vi "test_TCP_2_ Host.vi"() -> ()   [LabVIEW 2014]
panel:
  out "output array":string[](array[string])
  out "output_strCmd":string
  out "output_strAccum":string
  out "error out":errorcluster
  in  "stop":bool
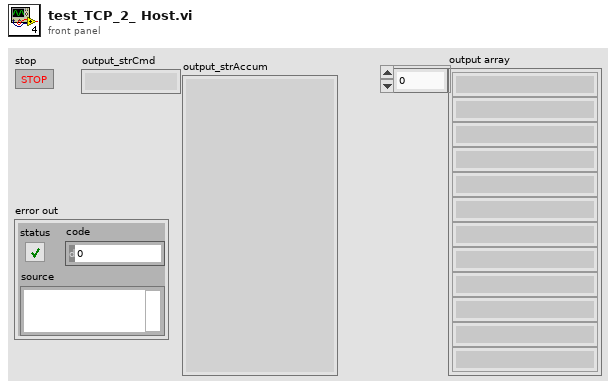
[diagram p1: front panel]
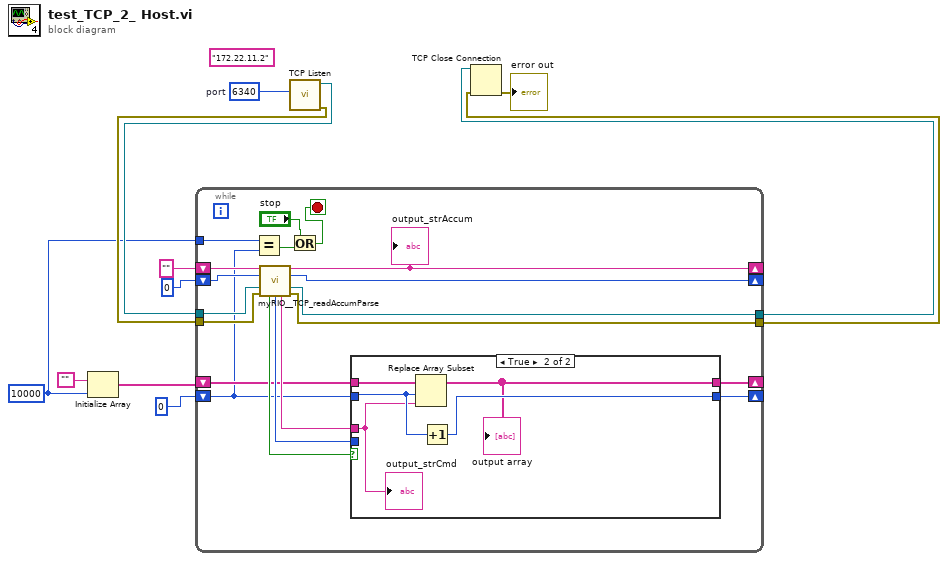
[diagram p0: block diagram]
diagram:
  w1 = 10000 ("dimension size")
  (unwired) "172.22.11.2" ("address")
  w8 = u16 6340  # port
  n1 = Initialize Array("", w1) -> (w2:string[])
  n2 = call <vilib>:"TCP Listen.vi"("port"=w8) -> ("error out"=w6:errorcluster, "connection ID"=w7:refnum<k5>)  [unwired: 6 in, 3 out]
  n3 = while {
    tunnel: w7 -> [w31]
    tunnel: [w28] -> w10
    shift-right: [w26] -> _
    shift-left: "" -> [w29]
    tunnel: w6 -> [w30]
    tunnel: [w27] -> w11
    shift-right: [w24] -> _
    shift-left: 0 -> [w25]
    shift-right: [w19] -> _
    shift-left: w2 -> [w20]
    shift-right: [w18] -> _
    shift-left: 0 -> [w13]
    tunnel: w1 -> [w14]
    stop <- w15 stop-if-true
    n4 = Equal?(x=w14, y=w13) -> (x = y?=w17:bool)
    n5 = call "myRIO__TCP_readAccumParse.vi"("input_strAccum"=w29, "input_count"=w25, "input_handle_TCP"=w31, "input_error"=w30) -> ("output_strAccum"=w26:string, "output_count"=w24:i32, "output_handle_TCP"=w28:refnum<k5>, "output_haveCmd"=w23:bool, "output_countCmd"=w22:i32, "output_strCmd"=w21:string, "output_error"=w27:errorcluster)  [unwired: 5 in]
    "output_strAccum" <- w26
    n6 = Or(x="stop", y=w17) -> (x .or. y?=w15:bool)
    n7 = case shown="True" w23 {
      tunnel: w22 -> [_ _]
      tunnel: w21 -> [_ w34]
      tunnel: w20 -> [w33 w38]
      tunnel: w13 -> [w32 w37]
      tunnel: [w33 w35] -> w19
      tunnel: [w32 w36] -> w18
      frame False {
      }
      frame True {
        n8 = Replace Array Subset(array=w38, new element=w34, index=w37) -> (w35:string[])
        "output array" <- w35
        n9 = Increment(x=w37) -> (x+1=w36:i32)
        "output_strCmd" <- w34
      }
    }
  }
  n10 = TCP Close Connection(connection ID=w10, error in (no error)=w11) -> (error out=→"error out":errorcluster)  [unwired: 2 out]
